vi "Parse_Register_Map.vi"(7 "Reg_Map_Bit_Name":string="HV_TRIM", 8 "Error In":errorcluster, 10 "Reg_Address_Data":T1={"Address"=81, "Data"=0} {"Address" format="%.0x"}, 11 "Reg_Map":string[][](array[string])=[["Reg Addr(0x00)", "7", "6", "5", "4", "3", "2", "1", "0"], ["0", "SPARE", "RF3_SH", "RF2_SH", "RF1_SH", "SPARE", "RF3_RFC", "RF2_RFC", "RF1_RFC"], ["1", "SPARE[7:0]", "", "", "", "", "", "", ""], ["2", "VVAR_EN", "LCM_EN", "RFC_SH", "SPARE", "VARACTOR[3:0]", "", "", ""], ["3", "SW_CTRL1_VIRTUAL[7:0]", "", "", "", "", "", "", ""], ["4", "SW_CTRL1_SWAP", "SW_CTRL1_RBSHIFT[2:0]", "", "", "SW_CTRL1_VSID[3:0]", "", "", ""], ["5", "REG_00_VIRTUAL_MASK[7:0]", "", "", "", "", "", "", ""], ["6", "LOCK_STATUS[1:0]", "", "CLK_DITHER", "FUSES_BURNED", "CLK_IDAC_CAL[3:0]", "", "", ""], ["7", "SPARE[2:0]", "", "", "ODFT_TRIM[4:0]", "", "", "", ""], ["8", "SPARE[2:0]", "", "", "HV_TRIM[4:0]", "", "", "", ""], ["9", "TEST_MUX[2:0]", "", "", "SPARE[1:0]", "", "MEMS_BG_TC[1:0]", "", "MEMSCP_RCM"], ["A", "CP_BOOST_OVRD_EN", "SPARE[2:0]", "", "", "PS_OFF_TIMER[1:0]", "", "PS_ON_TIMER[1:0]", ""], ["0", "", "", "", "", "", "", "", ""], ["D", "Reserved[1:0]", "", "WD_HI_EVENT_CNT[5:0]", "", "", "", "", ""], ["E", "VERSION_ID[7:0]", "", "", "", "", "", "", ""], ["F", "Reserved", "COUNT_200_LSB[6:0]", "", "", "", "", "", ""], ["10", "CLK_DIV2_EN", "Spare", "ODFT_EN", "HV_HYST[4:0]", "", "", "", ""], ["0", "", "", "", "", "", "", "", ""], ["12", "SHORT_FUSE", "FUSE_BURN", "STROBE_EN", "VIO_OK", "RTH[1:0]", "", "FUSE_LOAD_MAN_EN", "FUSE_LOAD"], ["13", "RR_ACK_EN", "Reserved", "ACK_POSITION[1:0]", "", "SuBUS_DRIVE_STRENGTH[3:0]", "", "", ""], ["14", "TM_IO_EN", "TM_IO_SEL", "SuBUS_OVS[1:0]", "", "Reserved[3:0]", "", "", ""], ["15", "Reserved[4:0]", "", "", "", "", "SuBUS_VERSION_PRESENT", "SuBUS_VOLTAGE", "SuBUS_FLAVOR_DEF"], ["16", "PROG_STROBE1_DUR[7:0]", "", "", "", "", "", "", ""], ["17", "PROG_STROBE0_DUR[7:0]", "", "", "", "", "", "", ""], ["18", "Reserved[2:0]", "", "", "EFUSE_SINGLE_ADDR_SEL[4:0]", "", "", "", ""], ["19", "POLL_ADR[4:0]", "", "", "", "", "POLL_BC[2:0]", "", ""], ["1A", "SOFTWARE_RESET", "Reserved[6:0]", "", "", "", "", "", ""], ["1B", "Reserved[7:0]", "", "", "", "", "", "", ""], ["1C", "PWR_MODE_1", "PWR_MODE_0", "TRIGGER_MASK[2:0]", "", "", "TRIGGER[2:0]", "", ""], ["1D", "PRODUCT_ID[7:0]", "", "", "", "", "", "", ""], ["1E", "MANUFACTURER_ID_LSB[7:0]", "", "", "", "", "", "", ""], ["1F", "MANUFACTURER_ID_MSB[7:0]", "", "", "", "", "", "", ""]]) -> (0 "Error Out":errorcluster, 1 "Length":u8, 2 "LSB":u8, 3 "MSB":u8)   [LabVIEW 2013]
uses:
  Controls/Reg_Address_Data.ctl
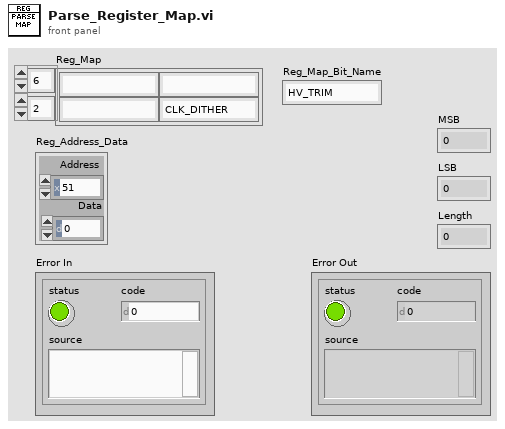
[diagram p1: front panel]
types:
  T1 = typedef "Reg_Address_Data.ctl" = cluster{"Address":u8, "Data":u8}
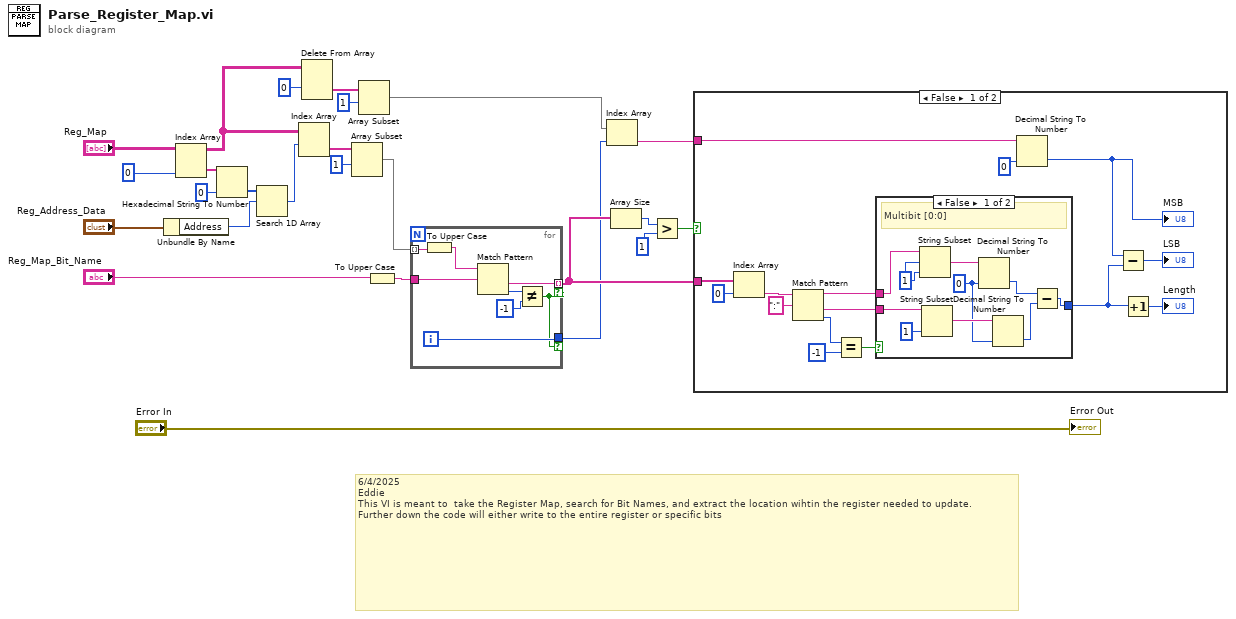
[diagram p0: block diagram]
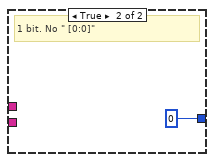
[diagram p2: hidden frame]
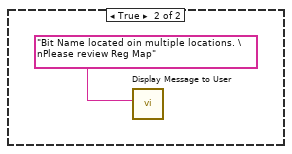
[diagram p3: hidden frame]
diagram:
  # "6/4/2025\nEddie\nThis VI is meant to  take the Register Map, search for Bit Names, and extract the location wihtin the register needed to update.\nFurther down the code will either write to the entire register or specific bits"
  n1 = Unbundle By Name("Reg_Address_Data") -> ("Address"=w19:u8)
  n2 = Index Array(array="Reg_Map", index (col)=0 ("disabled index (col)")) -> (element=w22:string[])  [unwired: 1 in]
  n3 = Hexadecimal String To Number(string=w22, default (0uL)=u8 0 ("default (0 U32)")) -> (number=w20:u8[])  [unwired: 1 in, 1 out]
  n4 = Search 1D Array(1D array=w20, element=w19) -> (index of element=w18:i32)  [unwired: 1 in]
  n5 = Index Array(array="Reg_Map", index (row)=w18) -> (element=w10:string[])  [unwired: 1 in]
  n6 = Delete From Array(array="Reg_Map", index (row)=0) -> (deleted portion=w7:string[])  [unwired: 2 in, 1 out]
  n7 = Array Subset(array=w10, index=1) -> (w5:string[])  [unwired: 1 in]
  n8 = Array Subset(array=w7, index=1) -> (w3:string[])  [unwired: 1 in]
  n9 = To Upper Case(1:"Reg_Map_Bit_Name") -> (0:w4:string)
  n10 = for {
    tunnel: w5 -> [w31] mode=indexing
    tunnel: w4 -> [w32]
    tunnel: [w27] -> w15 mode=indexing if=w25
    tunnel: [w26] -> w2 if=w25
    i -> [w26]
    n11 = To Upper Case(1:w31) -> (0:w30:string)
    n12 = Match Pattern(string=w30, regular expression=w32) -> (after substring=w27:string, offset past match=w29:i32)  [unwired: 1 in, 2 out]
    n13 = Not Equal?(x=w29, y=-1) -> (x != y?=w25:bool)
  }
  n14 = Index Array(array=w3, index=w2) -> (element=w1:string)
  n15 = Array Size(array=w15) -> (size(s)=w14:i32)
  n16 = Greater?(x=w14, y=1) -> (0:w12:bool)
  n17 = case shown="False" w12 {
    tunnel: w15 -> [w43 _]
    tunnel: w1 -> [w36 _]
    frame False {
      n18 = Index Array(array=w43, index=0) -> (element=w42:string)
      n19 = Match Pattern(string=w42, regular expression=":") -> (before substring=w45:string, after substring=w44:string, offset past match=w35:i32)  [unwired: 1 in, 1 out]
      n20 = Equal?(x=w35, y=-1) -> (x = y?=w33:bool)
      n21 = case shown="False" w33 {
        tunnel: w45 -> [w57 _]
        tunnel: w44 -> [w55 _]
        tunnel: [w49 u8 0] -> w39
        frame False {
          w50 = u8 0 ("default (0 I32)")
          w56 = 1 ("length (rest)")
          # "Multibit [0:0]"
          n22 = String Subset(string=w57, offset (0)=w56, length (rest)=w56) -> (substring=w53:string)
          n23 = String Subset(string=w55, length (rest)=1 ("length (rest)")) -> (substring=w52:string)  [unwired: 1 in]
          n24 = Decimal String To Number(string=w53, default (0L)=w50) -> (number=w48:u8)  [unwired: 1 in, 1 out]
          n25 = Decimal String To Number(string=w52, default (0L)=w50) -> (number=w51:u8)  [unwired: 1 in, 1 out]
          n26 = Subtract(x=w48, y=w51) -> (x-y=w49:u8)
        }
        frame True {
          # "1 bit. No \" [0:0]\""
        }
      }
      n27 = Decimal String To Number(string=w36, default (0L)=u8 0 ("default (0 I32)")) -> (number=w40:u8)  [unwired: 1 in, 1 out]
      "MSB" <- w40
      n28 = Subtract(x=w40, y=w39) -> (x-y=→"LSB":u8)
      n29 = Increment(x=w39) -> (x+1=→"Length":u8)
    }
    frame True {
      n30 = call "Display Message to User"("Message"="Bit Name located oin multiple locations. \nPlease review Reg Map") -> ()  [unwired: 9 in, 2 out]
    }
  }
  "Error Out" <- "Error In"
